vi "练习 2.vi"() -> ()   [LabVIEW 2021]
panel:
  in  "stop":bool
  in  "电压":dbl
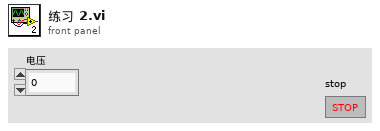
[diagram p1: front panel]
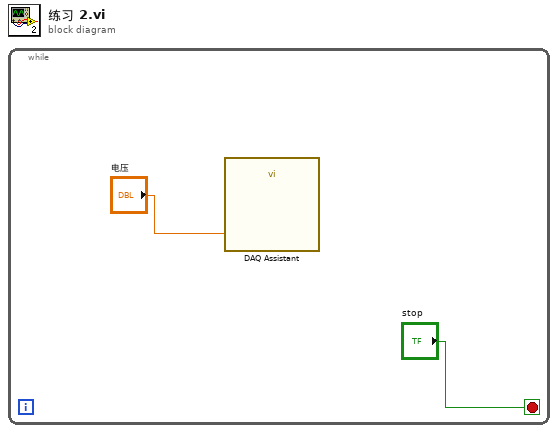
[diagram p0: block diagram]
diagram:
  n1 = while {
    stop <- "stop" stop-if-true
    n2 = call "DAQ Assistant"("data"="电压") -> ()  [unwired: 17 in, 2 out]
  }
